vi "Settings Panel.vi"() -> ()   [LabVIEW 2009, in "Scan Driver.lvclass"]
doc: "Main method of the Scan Driver class. Construct a new Scan Driver instance from the given options, or load and deserialize one from an XML file, or modify the last run scan. Configure the instance. Run the scan, and repeat it if more than one scan is requested."
uses:
  Scan Driver.lvclass
  Scanner List.ctl
  Reader List.ctl
  Scan Setup Mode.ctl
  Global/File Locations.vi
  Scan Driver.lvclass/Scan Driver.ctl
  File IO/File IO.lvclass
  Instruments/Utility Classes/Instrument/Instrument.lvclass
panel:
  in  "Use LCD?":bool
  in  "Based on Last Scan":bool=TRUE
  in  "Path":path
  in  "Scanner":T1=enum."Magnetic Field"
  in  "Reader":T2=enum."Photon Counter"
  in  "Scan Setup":T3
  out "Update UI":bool
  in  "Continue":bool
  out "error out":errorcluster
  in  "error in (no error)":errorcluster
  in  "exit":bool
  out "dispscan":string caption="Scan Settings"
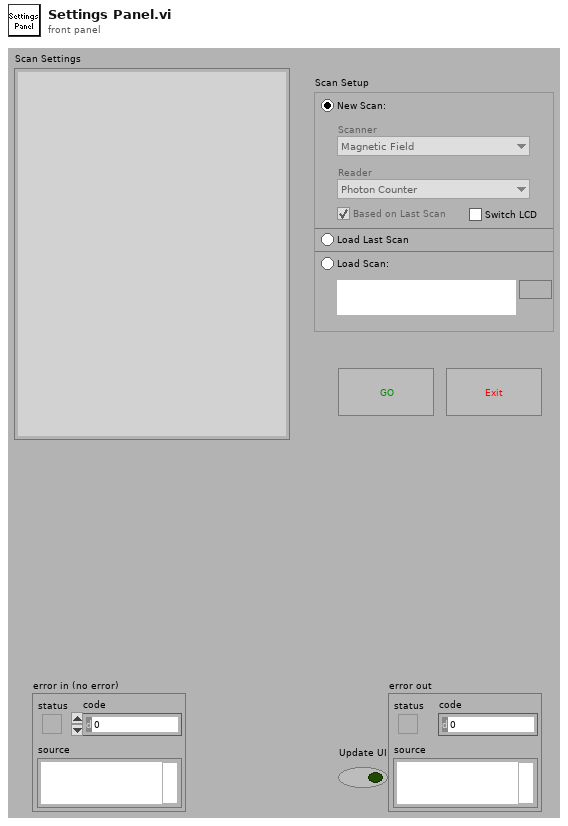
[diagram p1: front panel]
types:
  T1 = typedef "Scan Driver.lvclass/Scanner List.ctl" = enum16{"Wavelength", "Wavelength Digikröm", "Magnetic Field", "Continuous", "Pulse Gen Scan", "Pulse Gen Basic Scan", "Function Gen Scan", "Microwave Freq Scan", "Translation Stage Scan", "Dummy Scan", "Varian Magnet Scan", "Analog Output Scan"}
  T2 = typedef "Scan Driver.lvclass/Reader List.ctl" = enum16{"DAQmx Analog", "Dummy", "Lockin SR830", "Photon Counter"}
  T3 = typedef "Scan Driver.lvclass/Scan Setup Mode.ctl" = enum32{"New Scan", "Load Last Scan", "Load Scan:"}
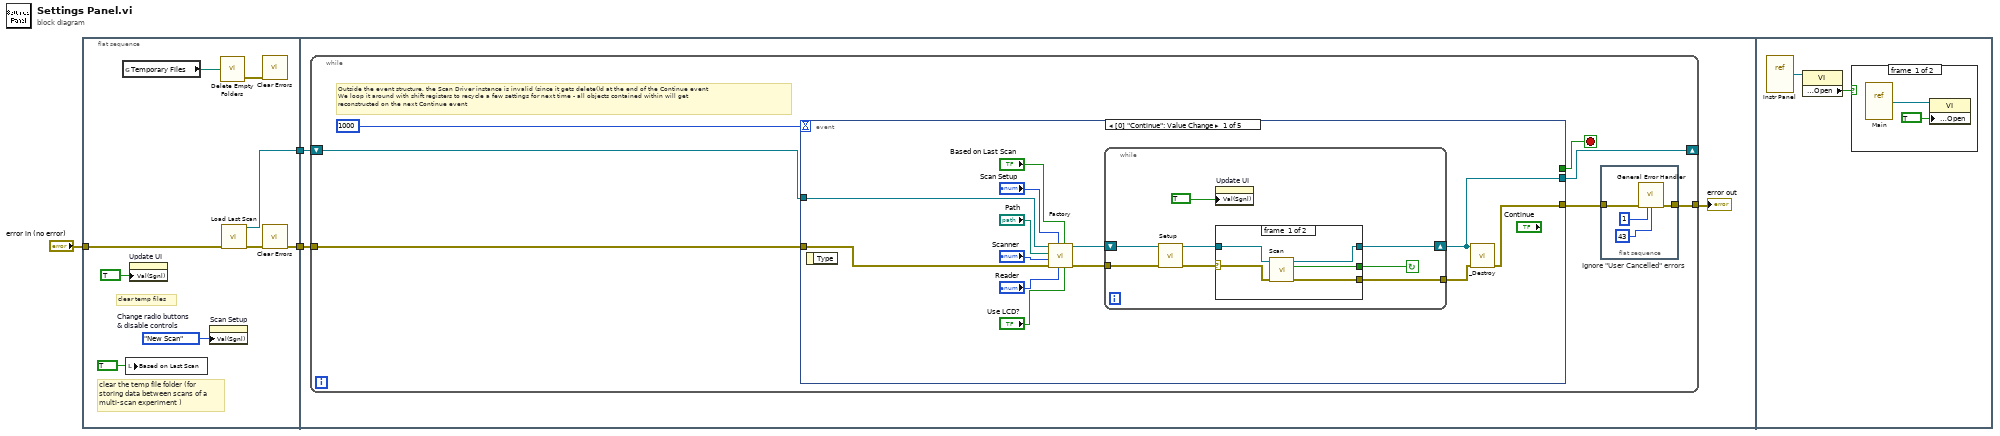
[diagram p0: block diagram]
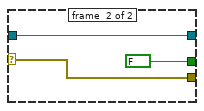
[diagram p2: hidden frame]
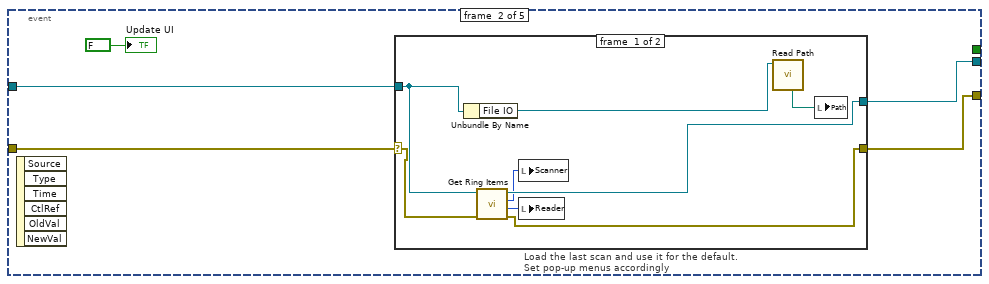
[diagram p3: hidden frame]
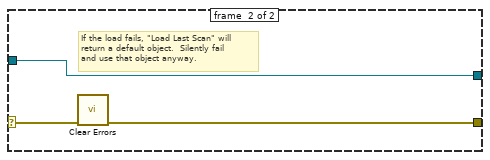
[diagram p4: hidden frame]
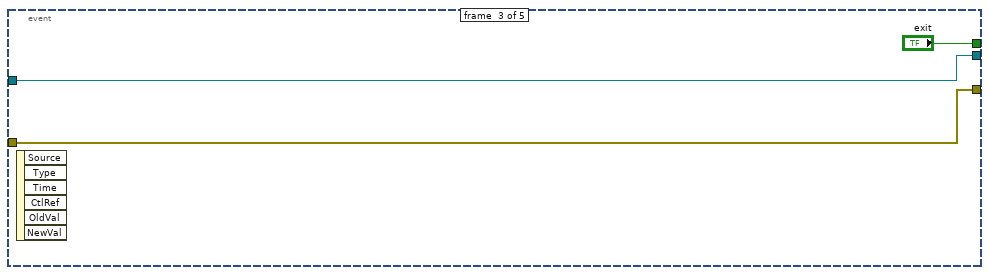
[diagram p5: hidden frame]
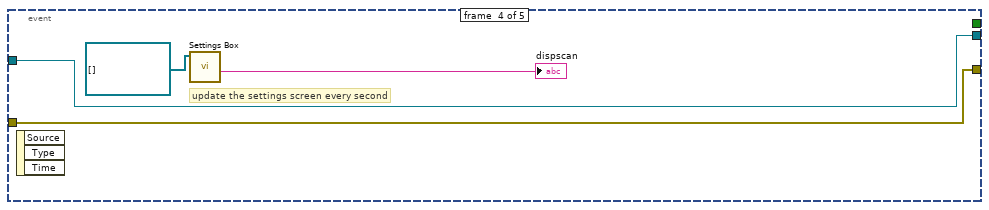
[diagram p6: hidden frame]
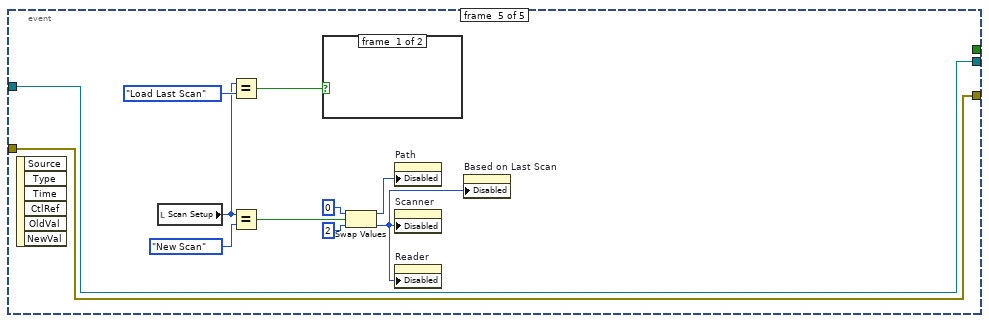
[diagram p7: hidden frame]
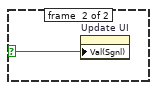
[diagram p8: hidden frame]
diagram:
  n1 = flat-sequence {
    tunnel: "error in (no error)" -> [w10]
    tunnel: [w4] -> w2
    tunnel: [w6] -> w1
    tunnel: w2 -> [w14]
    tunnel: w1 -> [w13]
    frame #0 {
      w8 = Scan_Setup_Mode."New Scan"  # Change radio buttons & disable controls
      # "clear the temp file folder (for storing data between scans of a multi-scan experiment )"
      # "clear temp files"
      n2 = global read "File Locations.vi" "Temporary Files"() -> (w12:path)
      n3 = local write "Based on Last Scan"(TRUE ("Based on Last Scan")) -> ()
      n4 = property on="Update UI" class="Bool (strict)"("Val(Sgnl)"=TRUE ("Value (Signaling)")) -> ()  [unwired: 2 in, 2 out]
      n5 = property on="Scan Setup" class="RadioBtnsControl (strict)"("Val(Sgnl)"=w8) -> ()  [unwired: 2 in, 2 out]
      n6 = call "Delete Empty Folders.vi"("dirpath"=w12) -> ("error out"=w11:errorcluster)  [unwired: 4 out]
      n7 = call "Load Last Scan.vi"("error in"=w10) -> ("error out"=w7:errorcluster, "Last Run Scan"=w6:refnum<class "Scan Driver.lvclass">)  [unwired: 9 out]
      n8 = call <vilib>:"Clear Errors.vi"("error in (no error)"=w11) -> ()  [unwired: 7 out]
      n9 = call <vilib>:"Clear Errors.vi"("error in (no error)"=w7) -> ("error out"=w4:errorcluster)  [unwired: 6 out]
    }
    frame #1 {
      n10 = while {
        shift-right: [w22] -> _
        shift-left: w13 -> [w17]
        tunnel: [w18] -> w15
        tunnel: w14 -> [w16]
        stop <- w21 stop-if-true
        # "Outside the event structure, the Scan Driver instance is invalid (since it gets delete()d at the end of the Continue event\nWe loop it around with shift registers to recycle a few settings for next time - all objects contained within will get\nreconstructed on the next Continue event"
        n11 = event shown="[0] \"Continue\": Value Change" {
          selector: _ -> [_ _ _ _ _]
          dyn-events: _ -> [_ _ _ _ _]
          timeout: 1000 -> [_ _ _ _ _]
          tunnel: [w37 w58 w73 w76 w86] -> w22
          tunnel: [w31 w60 w72 w75 w82] -> w19
          tunnel: w16 -> [w36 w59 w72 w75 w82]
          tunnel: [_ _ "exit" _ _] -> w21
          tunnel: w17 -> [w35 w57 w73 w76 w86]
          event #0 {
            n12 = event-data() -> ()  [unwired: 2 out]
            n13 = call "Factory.vi"("Use LCD?"="Use LCD?", "Recycle?"="Based on Last Scan", "Reader"="Reader", "Scan Setup Mode"="Scan Setup", "error in"=w36, "Scanner"="Scanner", "Path"="Path", "Recycle old Scan Driver in"=w35) -> ("error out"=w38:errorcluster, "Scan Driver out"=w39:refnum<class "Scan Driver.lvclass">)  [unwired: 2 out]
            n14 = while {
              tunnel: [w42] -> w30
              tunnel: w38 -> [w45]
              shift-right: [w41] -> w37
              shift-left: w39 -> [w46]
              stop <- w44 continue-if-true
              n15 = call-dynamic "Setup.vi"("error in (no error)"=w45, "Scan Driver in"=w46) -> ("error out"=w43:errorcluster, "Scan Driver out"=w47:refnum<class "Scan Driver.lvclass">)  [unwired: 8 out]
              n16 = property on="Update UI" class="Bool (strict)"("Val(Sgnl)"=TRUE ("Value (Signaling)")) -> ()  [unwired: 2 in, 2 out]
              n17 = case shown="No Error" w43 {
                selector: w43 -> [w49 w55]
                tunnel: w47 -> [w52 w54]
                tunnel: [w51 w54] -> w41
                tunnel: [w50 w55] -> w42
                tunnel: [w48 FALSE ("Again?")] -> w44
                frame #0 {
                  n18 = call "Scan.vi"("error in (no error)"=w49, "Scan Driver in"=w52) -> ("error out"=w50:errorcluster, "Again?"=w48:bool, "Scan Driver out"=w51:refnum<class "Scan Driver.lvclass">)  [unwired: 7 out]
                }
                frame #1 {
                }
              }
            }
            n19 = call-dynamic "_Destroy.vi"("error in (no error)"=w30, "Scan Driver in"=w37) -> ("error out"=w31:errorcluster)  [unwired: 9 out]
          }
          event #1 {
            n20 = event-data() -> ()  [unwired: 7 out]
            n21 = case "Load the last scan and use it for the default.  Set pop-up menus accordingly" shown="No Error" w59 {
              selector: w59 -> [w65 w71]
              tunnel: [w66 w69] -> w58
              tunnel: [w64 w70] -> w60
              tunnel: w57 -> [w63 w69]
              frame #0 {
                n22 = Unbundle By Name(w63) -> ("File IO"=w68:refnum<class "File IO.lvclass">)
                n23 = call "Get Ring Items.vi"("error in (no error)"=w65, "Scan Driver in"=w63) -> ("error out"=w64:errorcluster, "Reader"=w61:T2, "Scanner"=w62:T1, "Scan Driver out"=w66:refnum<class "Scan Driver.lvclass">)  [unwired: 6 out]
                n24 = local write "Scanner"(w62) -> ()
                n25 = local write "Reader"(w61) -> ()
                n26 = call-dynamic "Read Path.vi"("File IO.lvclass in"=w68) -> ("Settings Path"=w67:path)  [unwired: 1 in, 9 out]
                n27 = local write "Path"(w67) -> ()
              }
              frame #1 {
                # "If the load fails, \"Load Last Scan\" will\nreturn a default object.  Silently fail\nand use that object anyway."
                n28 = call <vilib>:"Clear Errors.vi"("error in (no error)"=w71) -> ("error out"=w70:errorcluster)  [unwired: 6 out]
              }
            }
            "Update UI" <- FALSE ("Update UI")
          }
          event #2 {
            n29 = event-data() -> ()  [unwired: 7 out]
          }
          event #3 {
            # "update the settings screen every second"
            n30 = event-data() -> ()  [unwired: 4 out]
            n31 = call "Settings Box.vi"("Instrument array"=refnum<class "Instrument.lvclass">[] []) -> ("statusbox"=→"dispscan":string)  [unwired: 1 in, 9 out]
          }
          event #4 {
            n32 = event-data() -> ()  [unwired: 7 out]
            n33 = local read "Scan Setup"() -> (w80:T3)
            n34 = Equal?(x=w80, y=Scan_Setup_Mode."Load Last Scan") -> (x = y?=w79:bool)
            n35 = Equal?(x=w80, y=Scan_Setup_Mode."New Scan") -> (x = y?=w85:bool)
            n36 = case shown="True" w79 {
              selector: w79 -> [_ w90]
              frame #0 {
              }
              frame #1 {
                n37 = property on="Update UI" class="Bool (strict)"("Val(Sgnl)"=w90) -> ()  [unwired: 2 in, 2 out]
              }
            }
            n38 = Swap Values(12:0 ("x"), 13:w85, 14:2 ("y")) -> (1:w89:i32, 3:w84:i32)
            n39 = property on="Path" class="Path"("Disabled"=w89) -> ()  [unwired: 2 in, 2 out]
            n40 = property on="Scanner" class="Enum (strict)"("Disabled"=w84) -> ()  [unwired: 2 in, 2 out]
            n41 = property on="Reader" class="Enum (strict)"("Disabled"=w84) -> ()  [unwired: 2 in, 2 out]
            n42 = property on="Based on Last Scan" class="Bool (strict)"("Disabled"=w84) -> ()  [unwired: 2 in, 2 out]
          }
        }
        n43 = flat-sequence "Ignore \"User Cancelled\" errors" {
          tunnel: w19 -> [w24]
          tunnel: [w23] -> w18
          frame #0 {
            n44 = call <vilib>:"General Error Handler.vi"("error in (no error)"=w24, "[exception action] (none:0)"=1, "[exception code]"=43) -> ("error out"=w23:errorcluster)  [unwired: 1 in, 11 out]
          }
        }
      }
      "error out" <- w15
    }
    frame #2 {
      n45 = vi-ref "Instr Panel.vi"() -> (w91:refnum<vi>)
      n46 = property class="VI"(reference=w91) -> ("Front Panel Window:Open"=w92:bool)  [unwired: 1 in, 2 out]
      n47 = case shown="False" w92 {
        frame #0 {
          n48 = vi-ref "Main.vi"() -> (w93:refnum<vi>)
          n49 = property class="VI"(reference=w93, "Front Panel Window:Open"=TRUE) -> ()  [unwired: 1 in, 2 out]
        }
        frame #1 {
        }
      }
    }
  }
